vi "send post-connection startup messages.vi"(11 "RT Queues":T1) -> (3 "RT Queues out":T1)   [LabVIEW 2018]
uses:
  Type Defs/Queues cluster.ctl
  ICL-LabVIEW_General/Message Scheduler/message scheduler.lvclass
  Queue VIs/En-queue RT comms element.vi
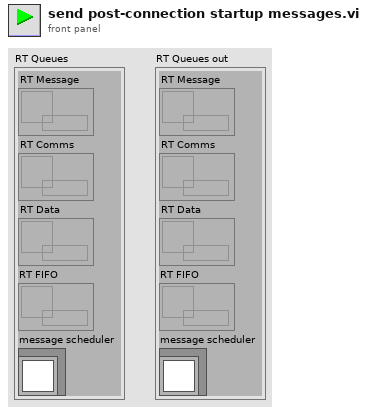
[diagram p1: front panel]
types:
  T1 = typedef "Queues cluster.ctl" = cluster{"RT Message":refnum<queue>, "RT Comms":refnum<queue>, "RT Data":refnum<queue>, "RT FIFO":refnum<queue>, "message scheduler":refnum<class "message scheduler.lvclass">}
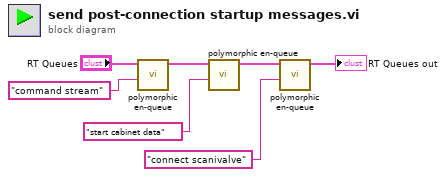
[diagram p0: block diagram]
diagram:
  n1 = call-poly "polymorphic en-queue.vi"("Message"="command stream", "RT Queues"="RT Queues") -> ("RT Queues out"=w4:T1)  [unwired: 9 in]
  n2 = call-poly "polymorphic en-queue.vi"("Message"="start cabinet data", "RT Queues"=w4) -> ("RT Queues out"=w3:T1)  [unwired: 9 in]
  n3 = call-poly "polymorphic en-queue.vi"("Message"="connect scanivalve", "RT Queues"=w3) -> ("RT Queues out"=→"RT Queues out":T1)  [unwired: 9 in]
